vi "GVSDV LOAD.vi"(8 "sData":string, 9 "nData":i32, 10 "pSPRef":refnum<vi>, 11 "sAction":string) -> (0 "nData_Out":i32, 1 "tWindow_Out":T1, 2 "pVIRef_Out":refnum<vi>, 3 "pSPRef_Out":refnum<vi>)   [LabVIEW 2013]
uses:
  GVSNew View Global.vi
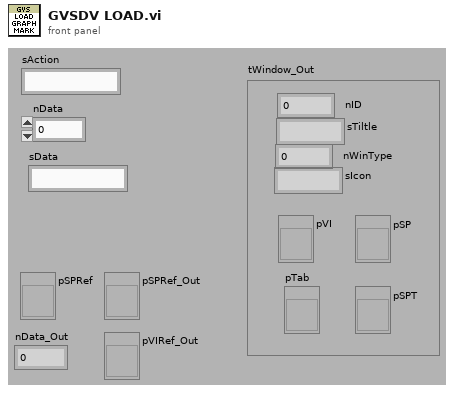
[diagram p1: front panel]
types:
  T1 = cluster{"nID":i32, "sTiltle":string, "pVI":refnum<vi>, "pSP":refnum<vi>, "pTab":refnum<vi>, "pSPT":refnum<vi>, "nWinType":i32, "sIcon":string}
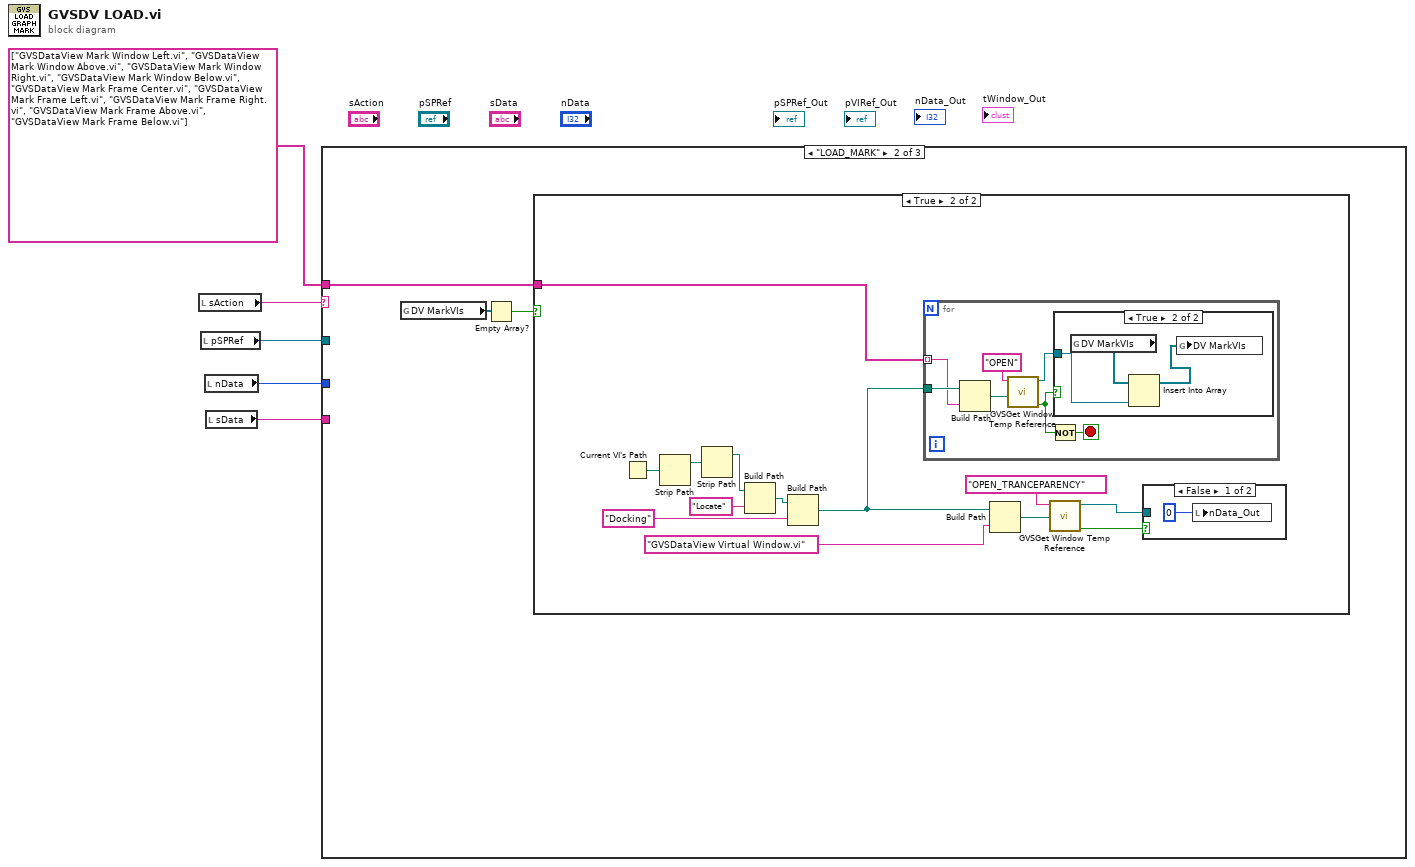
[diagram p0: block diagram]
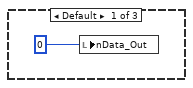
[diagram p2: hidden frame]
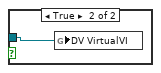
[diagram p4: hidden frame]
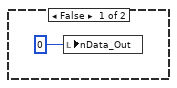
[diagram p5: hidden frame]
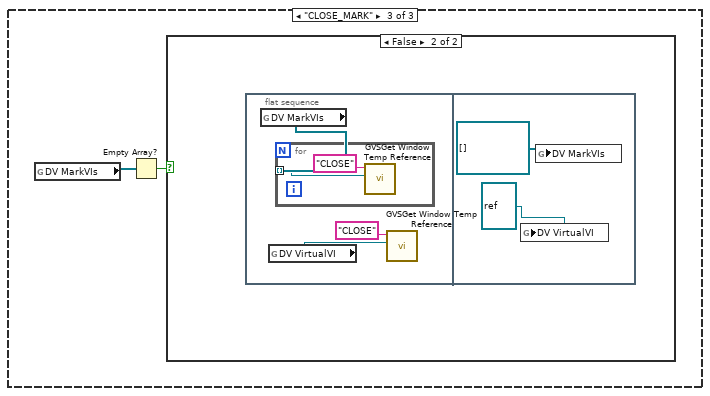
[diagram p6: hidden frame]
diagram:
  n1 = local read "sAction"() -> (w4:string)
  n2 = local read "pSPRef"() -> (w2:refnum<vi>)
  n3 = local read "nData"() -> (w1:i32)
  n4 = local read "sData"() -> (w3:string)
  n5 = case shown="\"LOAD_MARK\"" w4 {
    tunnel: string[] ["GVSDataView Mark Window Left.vi", "GVSDataView Mark Window Above.vi", "GVSDataView Mark Window Right.vi", "GVSDataView Mark Window Below.vi", "GVSDataView Mark Frame Center.vi", "GVSDataView Mark Frame Left.vi", "GVSDataView Mark Frame Right.vi", "GVSDataView Mark Frame Above.vi", "GVSDataView Mark Frame Below.vi"] -> [_ w9 _]
    tunnel: w3 -> [_ _ _]
    tunnel: w2 -> [_ _ _]
    tunnel: w1 -> [_ _ _]
    frame Default {
      n6 = local write "nData_Out"(0 ("nData_Out")) -> ()
    }
    frame "LOAD_MARK" {
      n7 = global read "GVSNew View Global.vi" "DV MarkVIs"() -> (w8:refnum<vi>[])
      n8 = Empty Array?(array=w8) -> (empty?=w7:bool)
      n9 = case shown="True" w7 {
        tunnel: w9 -> [_ w21]
        frame False {
        }
        frame True {
          n10 = Current VI's Path() -> (path=w19:path)
          n11 = Strip Path(path=w19) -> (stripped path=w18:path)  [unwired: 1 out]
          n12 = Strip Path(path=w18) -> (stripped path=w14:path)  [unwired: 1 out]
          n13 = Build Path(base path=w14, name or relative path="Locate") -> (appended path=w15:path)
          n14 = Build Path(base path=w15, name or relative path="Docking") -> (appended path=w20:path)
          n15 = for {
            tunnel: w20 -> [w31]
            tunnel: w21 -> [w30] mode=indexing
            stop <- w28 stop-if-true
            n16 = Build Path(base path=w31, name or relative path=w30) -> (appended path=w29:path)
            n17 = call "GVSGet Window Temp Reference.vi"("sVIFullName"=w29, "sAction"="OPEN") -> ("bResult"=w26:bool, "pVIRef_Out"=w25:refnum<vi>)  [unwired: 2 in, 6 out]
            n18 = Not(x=w26) -> (.not. x?=w28:bool)
            n19 = case shown="True" w26 {
              tunnel: w25 -> [_ w35]
              frame False {
                n20 = local write "nData_Out"(0 ("nData_Out")) -> ()
              }
              frame True {
                n21 = global read "GVSNew View Global.vi" "DV MarkVIs"() -> (w34:refnum<vi>[])
                n22 = Insert Into Array(array=w34, new element=w35) -> (w33:refnum<vi>[])  [unwired: 1 in]
                n23 = global write "GVSNew View Global.vi" "DV MarkVIs"(w33) -> ()
              }
            }
          }
          n24 = Build Path(base path=w20, name or relative path="GVSDataView Virtual Window.vi") -> (appended path=w13:path)
          n25 = call "GVSGet Window Temp Reference.vi"("sVIFullName"=w13, "sAction"="OPEN_TRANCEPARENCY") -> ("bResult"=w11:bool, "pVIRef_Out"=w10:refnum<vi>)  [unwired: 2 in, 6 out]
          n26 = case shown="False" w11 {
            tunnel: w10 -> [_ w24]
            frame False {
              n27 = local write "nData_Out"(0 ("nData_Out")) -> ()
            }
            frame True {
              n28 = global write "GVSNew View Global.vi" "DV VirtualVI"(w24) -> ()
            }
          }
        }
      }
    }
    frame "CLOSE_MARK" {
      n29 = global read "GVSNew View Global.vi" "DV MarkVIs"() -> (w36:refnum<vi>[])
      n30 = Empty Array?(array=w36) -> (empty?=w37:bool)
      n31 = case shown="False" w37 {
        frame True {
        }
        frame False {
          n32 = flat-sequence {
            frame #0 {
              n33 = global read "GVSNew View Global.vi" "DV MarkVIs"() -> (w39:refnum<vi>[])
              n34 = global read "GVSNew View Global.vi" "DV VirtualVI"() -> (w38:refnum<vi>)
              n35 = for {
                tunnel: w39 -> [w41] mode=indexing
                n36 = call "GVSGet Window Temp Reference.vi"("pVIRef_In"=w41, "sAction"="CLOSE") -> ()  [unwired: 5 in, 5 out]
              }
              n37 = call "GVSGet Window Temp Reference.vi"("pVIRef_In"=w38, "sAction"="CLOSE") -> ()  [unwired: 2 in, 8 out]
            }
            frame #1 {
              n38 = global write "GVSNew View Global.vi" "DV VirtualVI"(refnum<vi> refnum ("VIRef_Virtual")) -> ()
              n39 = global write "GVSNew View Global.vi" "DV MarkVIs"(refnum<vi>[] [] ("VIRef_Mark")) -> ()
            }
          }
        }
      }
    }
  }
